vi "Stop Condition - Saturation 2 (SubVI).vi"(8 "error in (no error)":errorcluster, 9 "Test RunTime":dbl, 10 "Time":dbl, 11 "Cluster in":T1 {"M Event" items=["Stop", "Running", "PID", "Up Limit", "Down Limit", "Load Limit"]; "Test Type" items=["Please Select", "Triaxial Shear", "Triaxial UU", "Shearbox", "Permeability", "Consolidation (Stepped Loading)/Swelling", "Saturation (Incremental)", "User Defined", "UCT", "Isotropic Consolidation", "Swelling Pressure"]; "Data"."Test Type" items=["Please Select", "Triaxial Shear", "Triaxial UU", "Shearbox", "Permeability", "Consolidation (Stepped Loading)/Swelling", "Saturation (Incremental)", "User Defined", "UCT", "Isotropic Consolidation", "Swelling Pressure"]}) -> (0 "error out":errorcluster, 1 "String":string, 2 "Boolean":bool, 3 "Cluster out":T1 {"M Event" items=["Stop", "Running", "PID", "Up Limit", "Down Limit", "Load Limit"]; "Test Type" items=["Please Select", "Triaxial Shear", "Triaxial UU", "Shearbox", "Permeability", "Consolidation (Stepped Loading)/Swelling", "Saturation (Incremental)", "User Defined", "UCT", "Isotropic Consolidation", "Swelling Pressure"]; "Data"."Test Type" items=["Please Select", "Triaxial Shear", "Triaxial UU", "Shearbox", "Permeability", "Consolidation (Stepped Loading)/Swelling", "Saturation (Incremental)", "User Defined", "UCT", "Isotropic Consolidation", "Swelling Pressure"]}, 4 "Delay":string, 5 "Enum":T10)   [LabVIEW 2019]
uses:
  Controls/RunTest - Data Structure.ctl
  Controls/Test Panel - Data Structure.ctl
  Controls/Station - Test Type.ctl
  <vilib>/Utility/miscctls.llb/LVRowAndColumnTypeDef.ctl
  Controls/RunTest - Calculate Data.ctl
  <vilib>/httpClient/ClientHandle.ctl
  Controls/RunTest - Start Condition.ctl
  Controls/RunTest - Stop Condition.ctl
  Controls/UDP - Event.ctl
  Controls/RunTest - State.ctl
  <vilib>/httpClient/LabVIEWHTTPClient.lvlib
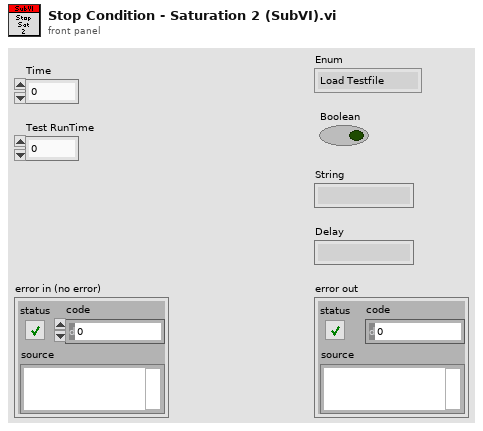
[diagram p1: front panel]
types:
  T1 = typedef "RunTest - Data Structure.ctl" = cluster{"Test Plan":string[], "PlanRow":i32, "Device Name":string[], "Timeout":i32, "Start?":bool, "Pause?":bool, "IP Address":string[], "LogRow":i32, "Logtype":u16, "Log Elapse":sgl, "Data":T2, "Stop log?":bool, "tdms":refnum<k34>, "Sensor Data":sgl[], "Start time":timestamp, "Prev Log Elapse":u32, "Plot":u16, "X-Axis":u16[], "Y-Axis":u16[], "XY":cluster{"X":dbl, "Y":dbl}[][], "End Stage?":bool, "1run":bool, "Condition":u16[], "Start Con":bool, "Log Con":bool, "Stop Con":bool, "Start Elapse":dbl, "Start Load":dbl, "Motor":i32, "StartRow":i32, "number log":i32, "Dir":bool, "Start time test":timestamp, "Auto":bool, "Check return?":bool, "Inv":cluster{"M":i32[], "Bool":bool[]}, "tdms temp":refnum<k34>, "Zero?":bool, "Plot Timer":dbl, "1st Run":bool, "TDMS Path":path, "MaxLoad":dbl, "Log Timer":sgl[], "Test Type":T3, "Log Sensor":string[], "Save?":bool, "1st Log":bool, "Y-Axis 2":u16[], "On Y-Axis 2":bool, "Decimal":u8[], "Init":cluster{"PWP TS":sgl, "Load TS":sgl, "Volume TS":sgl, "Disp TS":sgl, "CP":sgl, "Vol In":sgl, "Vol Out":sgl, "Load UCT":sgl, "Disp UCT":sgl, "PWP Sat":sgl, "CP Sat":sgl, "Volume IsoCons":sgl, "PWP IsoCons":sgl, "PWP TUU":sgl, "Load TUU":sgl, "Volume TUU":sgl, "Disp TUU":sgl, "Load Cons":sgl, "Disp Cons":sgl, "Volume Sat":sgl, "Vertical Load SB":sgl, "Vertical Disp SB":sgl, "H Disp SB":sgl, "H Load SB":sgl}, "Calc":T5, "Device Index":i32[], "Channel Index":i32[], "http ref":T6, "fileid":string, "Step Cons":cluster{"V Stress":sgl, "H Settlement":sgl}, "RunTest":bool, "Graph Last":i32, "Init?":bool, "Datalog":bool[], "Start":T7, "Stop":T8, "Running?":bool, "StartTime":dbl, "Log Prev Time":dbl, "KeyName":string[], "Test RunTime":dbl, "Log Prev Axial":dbl, "M Event":T9[], "Last Log":bool, "popup":bool, "PreStart UU":bool, "PreStart Sat":bool}
  T2 = typedef "Test Panel - Data Structure.ctl" = cluster{"Station":string, "Sample ID":string, "Job No":string, "Job Description":string, "Filename":string, "Test Type":T3, "Speciment No":string, "Depth":string, "Height":string, "Diameter/Length":string, "Weight":string, "Test Parameter":string, "Station[]":string[], "Edit Pos":T4, "Edit Pos Prev":T4, "Area":string, "Path":string}
  T3 = typedef "Station - Test Type.ctl" = u16
  T4 = typedef "LVRowAndColumnTypeDef.ctl" = cluster{"Row":i32, "Column":i32}
  T5 = typedef "RunTest - Calculate Data.ctl" = cluster{"TS":cluster{"Change PWP":sgl, "Change Vol":sgl, "Axial Load":sgl, "CiL":sgl, "Deviator":sgl, "Axial Strain":sgl, "MaxDeviator":sgl}, "TUU":cluster{"Change PWP":sgl, "Axial Load":sgl, "CiL":sgl, "Deviator":sgl, "Axial Strain":sgl, "MaxDeviator":sgl}, "Sat":cluster{"B Value":sgl, "PWP Diss":sgl, "CPP":sgl, "CV":sgl}, "Per":cluster{"Change Vol In":sgl, "Change Vol Out":sgl, "Mean Vol":sgl, "Gradient Pressure":sgl, "Outlet Flow":sgl, "Inlet Flow":sgl, "I X1":sgl, "I X2":sgl, "I Y1":sgl, "I Y2":sgl, "O X1":sgl, "O X2":sgl, "O Y1":sgl, "O Y2":sgl}, "Step Cons":cluster{"V Stress":sgl, "H Settlement":sgl, "Total H Settle":sgl, "Prev Total H":sgl}, "UCT":cluster{"ALC":sgl, "H Change":sgl, "Deviator":sgl, "Axial Strain":sgl, "V Stress":sgl, "MaxDeviator":sgl}, "ISO Cons":cluster{"CPP":sgl, "PWP Diss":sgl, "CV":sgl}, "SB":cluster{"Speci LenC":sgl, "Shear Strain":sgl, "H LC":sgl, "Normal Stress":sgl, "Shear Stress":sgl, "MaxShear":sgl}}
  T6 = typedef "LabVIEWHTTPClient.lvlib/ClientHandle.ctl" = refnum<k1>
  T7 = typedef "RunTest - Start Condition.ctl" = cluster{"Cons":cluster{"VS":dbl, "Delay":bool, "No Delay":dbl}, "Sat":cluster{"CP":dbl, "BP":dbl, "StartBP":bool, "Target CP":bool, "Target BP":bool}, "Iso":cluster{"Select":dbl, "BP":dbl, "IC2":dbl, "IC3":dbl, "IC4":dbl, ". IC6":bool, "IC6":dbl, "IC6-2":dbl, "Target":bool, "Time Cond":dbl, "Last PWP":dbl}, "TS":cluster{"SS":dbl, "Engage":bool, "ES":dbl, "LC":dbl, "PreStart":bool, "Trig SS":bool, "Drain":dbl}, "TUU":cluster{"SS":dbl, "Engage":bool, "ES":dbl, "LC":dbl, "PreStart":bool, "Trig SS":bool, "CP":dbl, "Delay Value":dbl, "Delay":bool, "CP PID":bool}, "UCT":cluster{"SS":dbl, "Engage":bool, "ES":dbl, "LC":dbl, "PreStart":bool, "Trig SS":bool}, "Enable?":bool, "SB":cluster{"SS":dbl, "Engage":bool, "ES":dbl, "LC":dbl, "PreStart":bool, "Trig SS":bool, "VS":dbl, "Delay Value":dbl, "Delay":bool, "VS PID":bool}, "Perm":cluster{"DP":dbl}}
  T8 = typedef "RunTest - Stop Condition.ctl" = cluster{"Cons":cluster{"Select":i32, "Disp":dbl, "Time":dbl, "Time2":dbl, "Disp 2":dbl, "Time Cond":dbl, "Last Disp":dbl, "Swell":bool}, "Sat":cluster{"Select":i32, "PP":dbl, "Time":dbl, "VC":dbl, "Time2":dbl, "Time Cond":dbl, "Last PP":dbl, ".B":bool, "B":dbl, "Last Vc":dbl, "Time Cond 2":dbl, "Time3":dbl, "Time Cond 3":dbl, "B Achieve":bool}, "Iso":cluster{"PP":dbl, "Time":dbl, "VC":dbl, "Time2":dbl, "Time Cond":dbl, "Last Vc":dbl, ".PP":bool, "Time Cond 2":dbl, "Select":i32}, "TS":cluster{"Axial":dbl, ".MaxDev":bool, "MaxDev Value":dbl, "Return":bool, "Reset":bool, "Prev Time":dbl, "PostStop Run":bool, "CP Stop":bool, "BP Stop":bool, "PostStop Trig":bool, "Reset Value":dbl, "BPTrig":bool, "CPTrig":bool, "VLCTrig":bool}, "TUU":cluster{"Axial":dbl, ".MaxDev":bool, "MaxDev Value":dbl, "Return":bool, "Reset":bool, "Prev Time":dbl, "PostStop Run":bool, "CP Stop":bool, "BP Stop":bool, "PostStop Trig":bool, "Reset Value":dbl, "BPTrig":bool, "CPTrig":bool, "VLCTrig":bool}, "UCT":cluster{"Axial":dbl, ".MaxDev":bool, "MaxDev Value":dbl, "Return":bool, "Reset":bool, "Prev Time":dbl, "PostStop Run":bool, "CP Stop":bool, "BP Stop":bool, "PostStop Trig":bool}, "Enable?":bool, "SB":cluster{"Shear":dbl, ".MaxShear":bool, "MaxShear Value":dbl, "Return":bool, "Reset":bool, "Prev Time":dbl, "PostStop Run":bool, "CP Stop":bool, "BP Stop":bool, "PostStop Trig":bool, "Reset Value":dbl, "BPTrig":bool, "CPTrig":bool, "VLCTrig":bool}, "Perm":cluster{"Max Time":bool, "Reset":bool, "PostStop Run":bool, "Ratio":bool, "Reset Value":dbl, "Time":dbl, "RatioTime":dbl, "RatioMore":dbl, "RatioLess":dbl, "Time Cond":dbl, "Time Cond 2":dbl, "Prev IF":dbl, "Prev OF":dbl, "PostStop Trig":bool, "BP Trig":bool, "DP Stop":bool, "BP Stop":bool, "CP Stop":bool, "CP Trig":bool}, "SP":cluster{".Max Time":bool, ".Time":bool, "Time":dbl, "MaxTime":dbl, "Time Cond":dbl, "Max Time Cond":dbl, "Stress":dbl}}
  T9 = typedef "UDP - Event.ctl" = u16
  T10 = typedef "RunTest - State.ctl" = enum16{"Load Testfile", "Notifier", "Init", "Idle", "Load", "Read DB", "Run", "Pause", "Stop", "Check Start", "Check Stop", "Check Post Stop", "Check Log", "EndStage", "Data View", "Display", "Graph", "Graph Old", "Close", "Stop PID", "Check Limit", "Auto", "Up", "Log", "Zero", "Machine Control", "Save Report"}
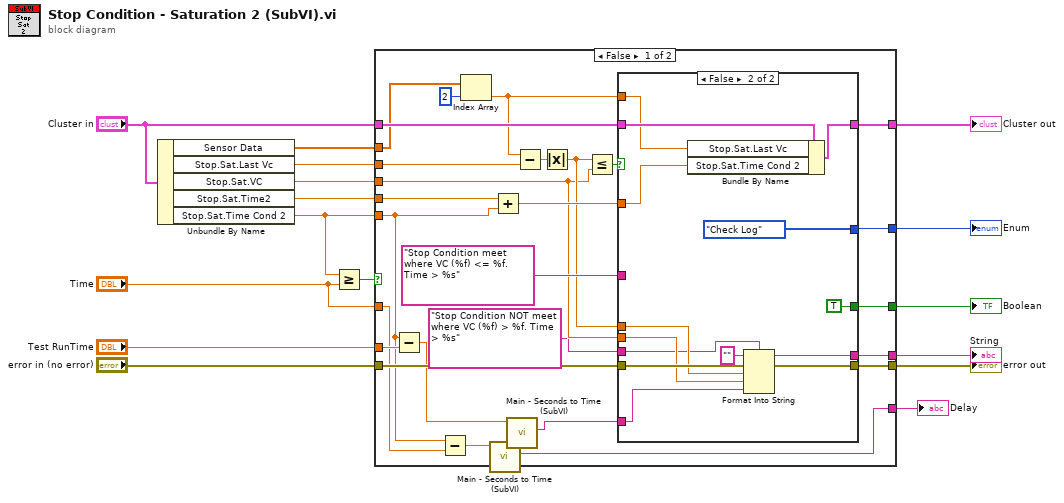
[diagram p0: block diagram]
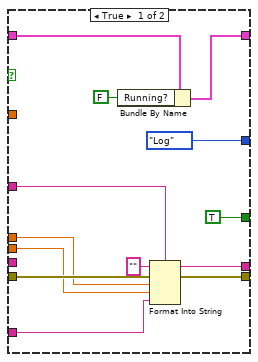
[diagram p2: hidden frame]
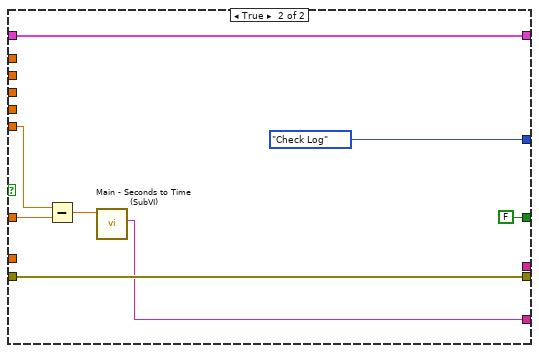
[diagram p3: hidden frame]
diagram:
  n1 = Unbundle By Name("Cluster in") -> ("Sensor Data"=w11:sgl[], "Stop.Sat.Last Vc"=w12:dbl, "Stop.Sat.VC"=w13:dbl, "Stop.Sat.Time2"=w14:dbl, "Stop.Sat.Time Cond 2"=w15:dbl)
  n2 = Greater Or Equal?(x=w15, y="Time") -> (x >= y?=w3:bool)
  n3 = case shown="False" w3 {
    tunnel: [w29 w77] -> w1
    tunnel: "error in (no error)" -> [w30 w77]
    tunnel: [w41 w76] -> w2
    tunnel: "Cluster in" -> [w40 w76]
    tunnel: w12 -> [w37 _]
    tunnel: w13 -> [w25 _]
    tunnel: w14 -> [w39 _]
    tunnel: w15 -> [w19 w72]
    tunnel: [w42 RunTest_-_State."Check Log"] -> w4
    tunnel: w11 -> [w34 _]
    tunnel: [w28 _] -> w6
    tunnel: [w27 FALSE] -> w7
    tunnel: "Time" -> [w18 w71]
    tunnel: "Test RunTime" -> [w24 _]
    tunnel: [w17 w70] -> w16
    frame False {
      n4 = Subtract(x=w19, y=w24) -> (x-y=w23:dbl)
      n5 = Subtract(x=w19, y=w18) -> (x-y=w20:dbl)
      n6 = Index Array(array=w34, index=2) -> (element=w33:sgl)
      n7 = call "Main - Seconds to Time (SubVI).vi"("Seconds"=w20) -> ("Time string"=w17:string)  [unwired: 9 in, 1 out]
      n8 = Add(x=w39, y=w19) -> (x+y=w38:dbl)
      n9 = call "Main - Seconds to Time (SubVI).vi"("Seconds"=w23) -> ("Time string"=w21:string)  [unwired: 9 in, 1 out]
      n10 = Subtract(x=w33, y=w37) -> (x-y=w36:dbl)
      n11 = Absolute Value(x=w36) -> (abs(x)=w26:dbl)
      n12 = Less Or Equal?(x=w26, y=w25) -> (x <= y?=w35:bool)
      n13 = case shown="False" w35 {
        tunnel: [RunTest_-_State."Log" RunTest_-_State."Check Log"] -> w42
        tunnel: [w54 w68] -> w41
        tunnel: w40 -> [w53 w67]
        tunnel: w38 -> [_ w66]
        tunnel: w33 -> [_ w65]
        tunnel: "Stop Condition meet where VC (%f) <= %f. Time > %s" -> [w51 _]
        tunnel: w30 -> [w49 w61]
        tunnel: [w48 w62] -> w29
        tunnel: [w47 w56] -> w28
        tunnel: [TRUE TRUE] -> w27
        tunnel: w21 -> [w45 w58]
        tunnel: w26 -> [w44 w60]
        tunnel: w25 -> [w43 w59]
        tunnel: "Stop Condition NOT meet where VC (%f) > %f. Time > %s" -> [_ w57]
        frame True {
          n14 = Bundle By Name(cluster=w53, "Running?"=FALSE) -> (w54:T1)
          n15 = Format Into String(format string=w51, initial string="", error in=w49, w44, w43, w45) -> (resulting string=w47:string, error out=w48:errorcluster)
        }
        frame False {
          n16 = Bundle By Name(cluster=w67, "Stop.Sat.Last Vc"=w65, "Stop.Sat.Time Cond 2"=w66) -> (w68:T1)
          n17 = Format Into String(format string=w57, initial string="", error in=w61, w60, w59, w58) -> (resulting string=w56:string, error out=w62:errorcluster)
        }
      }
    }
    frame True {
      n18 = Subtract(x=w72, y=w71) -> (x-y=w73:dbl)
      n19 = call "Main - Seconds to Time (SubVI).vi"("Seconds"=w73) -> ("Time string"=w70:string)  [unwired: 9 in, 1 out]
    }
  }
  "Delay" <- w16
  "Boolean" <- w7
  "String" <- w6
  "Enum" <- w4
  "Cluster out" <- w2
  "error out" <- w1
